vi "Populate_Item_List.vi"(8 "error in (no error)":errorcluster, 10 "TreeRef":refnum<vi>, 11 "object in":refnum<class "WebBrowser_Mgmt.lvclass">) -> (0 "error out":errorcluster, 3 "object out":refnum<class "WebBrowser_Mgmt.lvclass">)   [LabVIEW 2016, in "WebBrowser_Mgmt.lvclass"]
uses:
  WebBrowser_Mgmt.lvclass
  Crypter/Crypter.lvclass
  Crypter/Crypter.lvclass/Crypter.ctl
  WebBrowser_Mgmt.lvclass/WebBrowser_Mgmt.ctl
  Folder_Mgmt/Folder_Mgmt.lvclass
panel:
  out "Actual item tags (no duplicates)":string[](array[string])
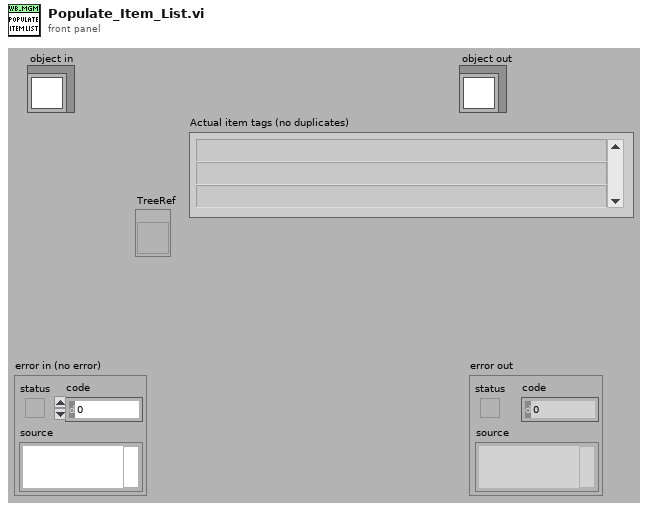
[diagram p1: front panel]
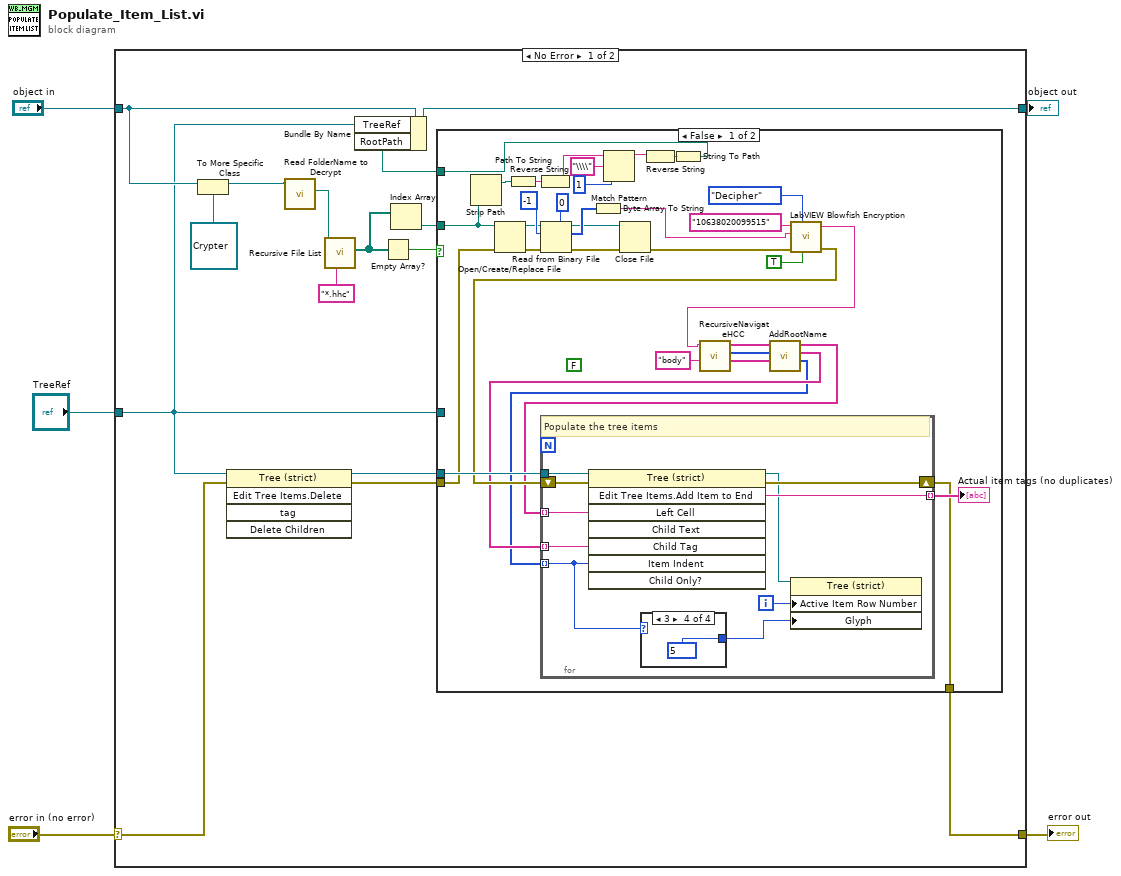
[diagram p0: block diagram]
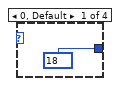
[diagram p2: hidden frame]
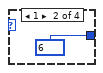
[diagram p3: hidden frame]
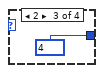
[diagram p4: hidden frame]
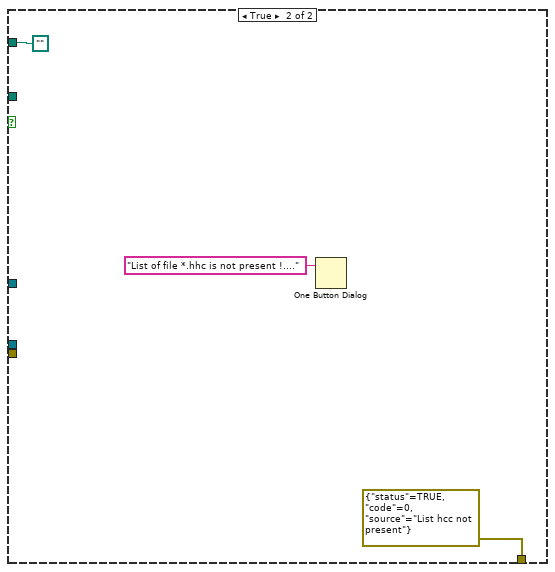
[diagram p5: hidden frame]
diagram:
  n1 = case shown="No Error" "error in (no error)" {
    selector: "error in (no error)" -> [w11 w73]
    tunnel: [w9 w73] -> w4
    tunnel: [w8 w72] -> w2
    tunnel: "object in" -> [w19 w72]
    tunnel: "TreeRef" -> [w7 _]
    frame No Error {
      n2 = To More Specific Class(target class=refnum<class "Crypter.lvclass"> refnum ("Crypter"), reference=w19) -> (specific class reference=w18:refnum<class "Crypter.lvclass">)  [unwired: 1 in, 1 out]
      n3 = invoke class="Tree (strict)" method="Edit Tree Items.Delete"(reference=w7, error in=w11) -> (reference out=w12:refnum<vi>, error out=w10:errorcluster)  [unwired: 3 in, 3 out]
      n4 = call "Read FolderName to Decrypt.vi"("Crypter in"=w18) -> ("FolderName to Decrypt"=w16:path)  [unwired: 8 in, 2 out]
      n5 = call <vilib>:"Recursive File List.vi"("pattern"="*.hhc" ("name or relative path"), "Folder Path"=w16) -> ("All Files in Dir"=w14:path[])  [unwired: 5 in, 4 out]
      n6 = Empty Array?(array=w14) -> (empty?=w15:bool)
      n7 = Index Array(array=w14) -> (element=w13:path)  [unwired: 1 in]
      n8 = case shown="False" w15 {
        tunnel: w7 -> [_ _]
        tunnel: w13 -> [w37 _]
        tunnel: w12 -> [w53 _]
        tunnel: w10 -> [w41 _]
        tunnel: [w51 errorcluster {"status"=TRUE, "code"=0, "source"="List hcc not present"} ("error out")] -> w9
        tunnel: [w28 path ""] -> w6
        frame False {
          (unwired) FALSE ("advisory dialog? (display:T)")
          n9 = Strip Path(path=w37) -> (stripped path=w36:path)  [unwired: 1 out]
          n10 = Open/Create/Replace File(file path (use dialog)=w37, error in=w41) -> (refnum out=w43:refnum<file>, error out=w45:errorcluster)  [unwired: 4 in, 1 out]
          n11 = Path To String(path=w36) -> (string=w35:string)
          n12 = Reverse String(1:w35) -> (0:w33:string)
          n13 = Read from Binary File(5:u8 0, 8:w45, 10:-1 ("count (1)"), 11:w43) -> (0:w44:errorcluster, 2:w46:u8[], 3:w42:refnum<file>)  [unwired: 2 in, 1 out]
          n14 = Byte Array To String(unsigned byte array=w46) -> (string=w34:string)
          n15 = Match Pattern(string=w33, regular expression="\\\\", offset (0)=1) -> (before substring=w30:string)  [unwired: 3 out]
          n16 = Close File(refnum=w42, error in=w44) -> (error out=w40:errorcluster)  [unwired: 1 out]
          n17 = Reverse String(1:w30) -> (0:w29:string)
          n18 = String To Path(string=w29) -> (path=w28:path)
          n19 = call "LabVIEW Blowfish Encryption.vi"("Password"="10638020099515", "Enc/Dec"=enum16{"Encipher", "Decipher"}."Decipher", "Input Text"=w34, "Output As ASCII\nfor email Transmission"=TRUE ("Output As ASCII\nfor email Transmission"), "error in (no error)"=w40) -> ("Output text"=w38:string, "error out"=w39:errorcluster)  [unwired: 1 in, 1 out]
          n20 = call "RecursiveNavigateHCC.vi"("SearchingFor"="body", "data"=w38) -> ("ItemTags"=w25:string[], "Ident"=w26:i32[], "ItemNames"=w27:string[])  [unwired: 7 in]
          n21 = call "AddRootName.vi"("ItemTags"=w25, "Ident"=w26, "ItemNames"=w27) -> ("ItemIdents"=w22:i32[], "ChildTags"=w24:string[], "LeftCellStrings"=w23:string[])  [unwired: 6 in]
          n22 = for {
            tunnel: w23 -> [w62] mode=indexing
            tunnel: [w60] -> w52 mode=indexing
            tunnel: w24 -> [w61] mode=indexing
            tunnel: w22 -> [w57] mode=indexing
            shift-right: [w63] -> w51
            shift-left: w39 -> [w64]
            tunnel: w53 -> [w59]
            i -> [w56]
            # "Populate the tree items"
            n23 = invoke on="Invoke Node" class="Tree (strict)" method="Edit Tree Items.Add Item to End"(reference=w59, error in=w64, "Left Cell"=w62, "Child Tag"=w61, "Item Indent"=w57) -> (reference out=w58:refnum<vi>, error out=w63:errorcluster, "Edit Tree Items:Add Item to End"=w60:string)  [unwired: 3 in, 5 out]
            n24 = case shown="3" w57 {
              tunnel: [18 ("Listbox Symbol Ring Constant") 6 ("Listbox Symbol Ring Constant") 4 ("Listbox Symbol Ring Constant") 5 ("Listbox Symbol Ring Constant")] -> w55
              frame 0, Default {
              }
              frame 1 {
              }
              frame 2 {
              }
              frame 3 {
              }
            }
            n25 = property class="Tree (strict)"(reference=w58, "Active Item Row Number"=w56, "Glyph"=w55) -> ()  [unwired: 1 in, 2 out]
          }
          "Actual item tags (no duplicates)" <- w52
        }
        frame True {
          n26 = One Button Dialog(message="List of file *.hhc is not present !....") -> ()  [unwired: 1 in, 1 out]
        }
      }
      n27 = Bundle By Name(cluster=w19, "TreeRef"=w7, "RootPath"=w6) -> (w8:refnum<class "WebBrowser_Mgmt.lvclass">)
    }
    frame Error {
    }
  }
  "error out" <- w4
  "object out" <- w2
